vi "Configure Measurement.vi"(0 "VISA resource name":refnum<visa-resource-name>, 1 "Rate (0: Slow)":i32(ring) items=["Slow", "Mid", "Fast"], 5 "Function (0: DC Volts)":i32(ring) items=["DC Volts", "AC Volts", "DC+AC Volts", "DC Current", "AC Current", "DC+AC Current", "2-Wire Resistance", "4-Wire Resistance", "Frequency", "Period", "Continuity", "Diode", "Temperature", "Capacitance"], 7 "Auto Range (T:Enable)":bool=TRUE, 9 "Manual Range (1.0)":dbl=1.0, 11 "error in (no error)":errorcluster, 12 "Threshold (10)":i32=10 min=0 max=1000 step=1) -> (4 "VISA resource name out":refnum<visa-resource-name>, 15 "error out":errorcluster)   [LabVIEW 2021, in "GWInstek  GDM8351.lvlib"]
doc: "Configures the measurement function, rate, and range on the instrument."
uses:
  <instrlib>/GWInstek  GDM8351/GWInstek  GDM8351.lvlib
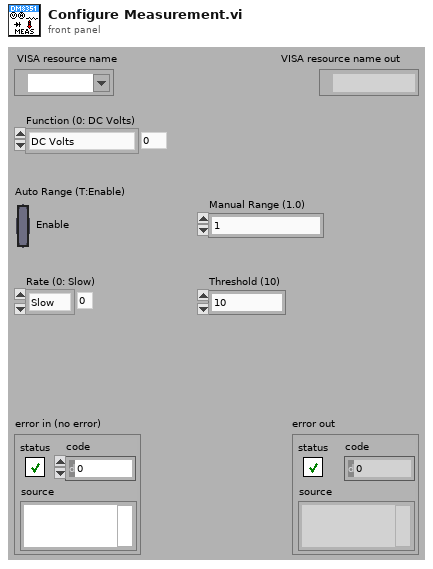
[diagram p1: front panel]
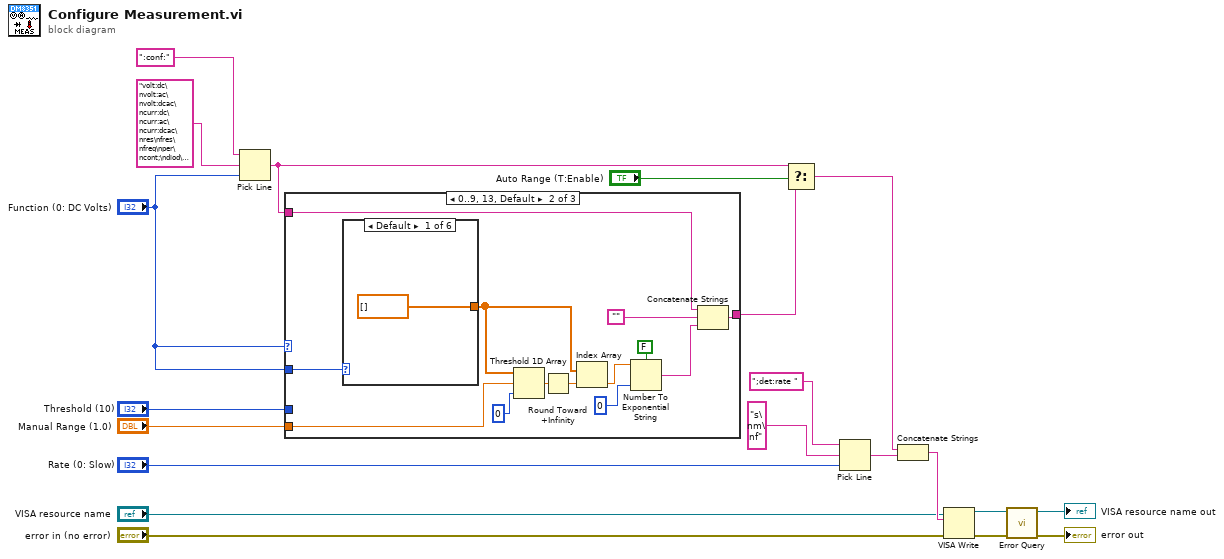
[diagram p0: block diagram]
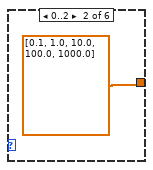
[diagram p3: hidden frame]
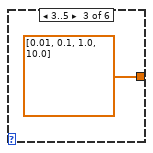
[diagram p4: hidden frame]
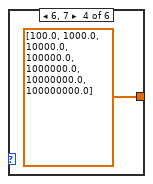
[diagram p5: hidden frame]
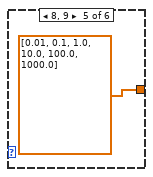
[diagram p6: hidden frame]
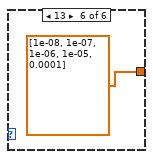
[diagram p7: hidden frame]
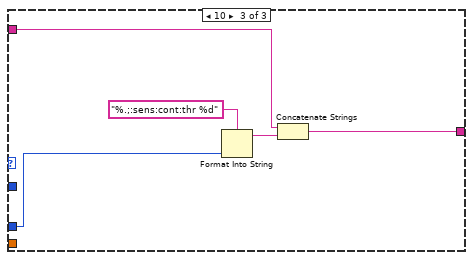
[diagram p8: hidden frame]
diagram:
  n1 = Pick Line(string ("")=":conf:", multi-line string="volt:dc\nvolt:ac\nvolt:dcac\ncurr:dc\ncurr:ac\ncurr:dcac\nres\nfres\nfreq\nper\ncont;\ndiod\ntemp:tco\ncap", line index="Function (0: DC Volts)") -> (output string=w5:string)
  n2 = case shown="0..9, 13, Default" "Function (0: DC Volts)" {
    tunnel: "Function (0: DC Volts)" -> [_ w27 _]
    tunnel: w5 -> [w21 w26 w43]
    tunnel: [w21 w28 w42] -> w4
    tunnel: "Threshold (10)" -> [_ _ w41]
    tunnel: "Manual Range (1.0)" -> [_ w23 _]
    frame 11, 12 {
    }
    frame 0..9, 13, Default {
      n3 = case shown="Default" w27 {
        tunnel: [dbl[] [] dbl[] [0.1, 1.0, 10.0, 100.0, 1000.0] dbl[] [0.01, 0.1, 1.0, 10.0] dbl[] [100.0, 1000.0, 10000.0, 100000.0, 1000000.0, 10000000.0, 100000000.0] dbl[] [0.01, 0.1, 1.0, 10.0, 100.0, 1000.0] dbl[] [1e-08, 1e-07, 1e-06, 1e-05, 0.0001]] -> w31
        frame Default {
        }
        frame 0..2 {
        }
        frame 3..5 {
        }
        frame 6, 7 {
        }
        frame 8, 9 {
        }
        frame 13 {
        }
      }
      n4 = Threshold 1D Array(1:0 ("start index (0)"), 2:w23, 3:w31) -> (0:w33:dbl)
      n5 = Round Toward +Infinity(x=w33) -> (ceil(x): smallest int >= x=w32:dbl)
      n6 = Index Array(array=w31, index=w32) -> (element=w30:dbl)
      n7 = Number To Exponential String(number=w30, precision (6)=i16 0, 1:FALSE ("use system decimal point (T)")) -> (E-format string=w24:string)  [unwired: 1 in]
      n8 = Concatenate Strings(w26, "" ("string"), w24) -> (w28:string)
    }
    frame 10 {
      n9 = Format Into String(format string="%.;:sens:cont:thr %d", w41) -> (resulting string=w44:string)  [unwired: 2 in, 1 out]
      n10 = Concatenate Strings(w43, w44) -> (w42:string)
    }
  }
  n11 = Select(t=w5, s="Auto Range (T:Enable)", f=w4) -> (s? t:f=w3:string)
  n12 = Pick Line(string ("")=";det:rate ", multi-line string="s\nm\nf", line index="Rate (0: Slow)") -> (output string=w13:string)
  n13 = Concatenate Strings(w3, w13) -> (w12:string)
  n14 = VISA Write(VISA resource name="VISA resource name", write buffer=w12, error in (no error)="error in (no error)") -> (VISA resource name out=w11:refnum<visa-resource-name>, error out=w10:errorcluster)  [unwired: 1 out]
  n15 = call <instrlib>:"Error Query.vi"("error in (no error)"=w10, "VISA resource name"=w11) -> ("error out"=→"error out":errorcluster, "VISA resource name out"=→"VISA resource name out":refnum<visa-resource-name>)  [unwired: 6 in, 2 out]
